vi "IO_Driver18v7.vi"(10 "Inputs":T3, 11 "Reply In":string) -> (0 "Tx Buf Out":string, 2 "Outputs":T2)   [LabVIEW 2024]
uses:
  Control Definitions/Def_Status18v7.ctl
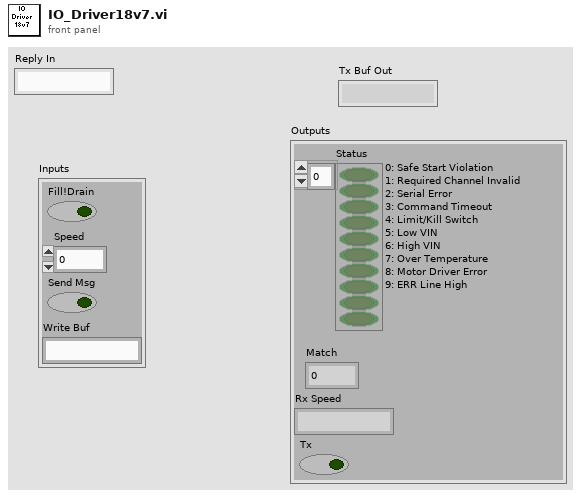
[diagram p1: front panel]
types:
  T1 = typedef "Def_Status18v7.ctl" = bool[]
  T2 = cluster{"Status":T1, "Match":i32, "Rx Speed":string, "Tx":bool}
  T3 = cluster{"Fill!Drain":bool, "Speed":i16, "Send Msg":bool, "Write Buf":string}
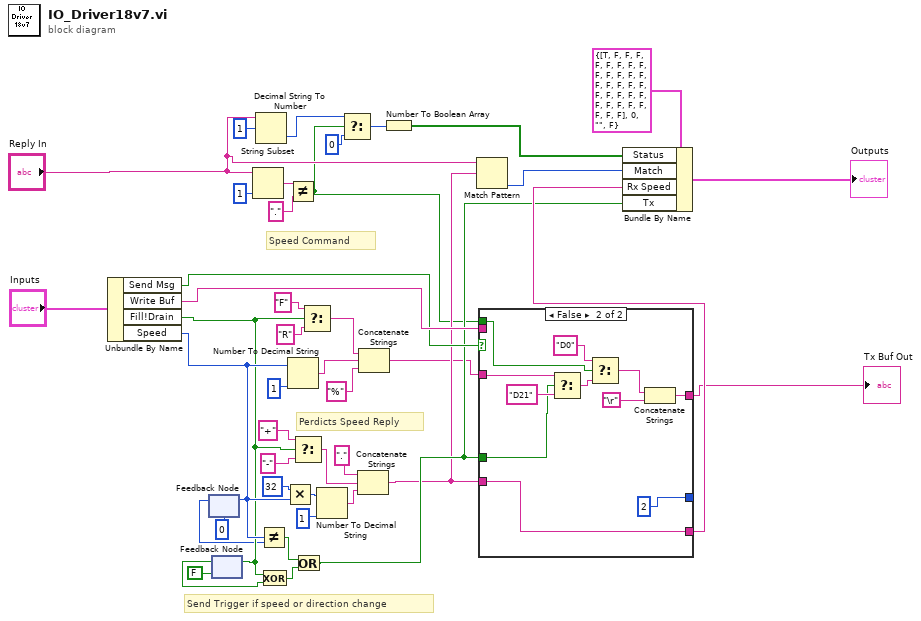
[diagram p0: block diagram]
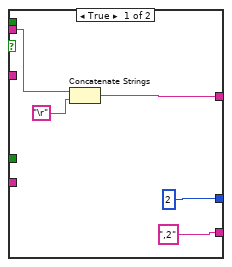
[diagram p2: hidden frame]
diagram:
  # "Send Trigger if speed or direction change"
  # "Speed Command"
  # "Perdicts Speed Reply"
  n1 = Unbundle By Name("Inputs") -> ("Send Msg"=w39:bool, "Write Buf"=w40:string, "Fill!Drain"=w41:bool, "Speed"=w42:i16)
  n2 = feedback #1(i16 0 ("Speed")) -> (w12:i16)
  n3 = feedback-in #1(w42) -> ()
  n4 = feedback #2(FALSE ("Fill!Drain")) -> (w20:bool)
  n5 = feedback-in #2(w41) -> ()
  n6 = String Subset(string="Reply In", length (rest)=1 ("length (rest)")) -> (substring=w25:string)  [unwired: 1 in]
  n7 = Decimal String To Number(string="Reply In", offset=1) -> (number=w28:i32)  [unwired: 1 in, 1 out]
  n8 = Not Equal?(x=w42, y=w12) -> (x != y?=w21:bool)
  n9 = Exclusive Or(1:w20, 2:w41) -> (0:w22:bool)
  n10 = Multiply(x=32, y=w42) -> (x*y=w7:i32)
  n11 = Not Equal?(x=w25, y=".") -> (x != y?=w30:bool)
  n12 = Number To Decimal String(number=w42, width (-)=i16 1) -> (decimal integer string=w17:string)
  n13 = Select(t="+", s=w41, f="-") -> (s? t:f=w9:string)
  n14 = Or(x=w21, y=w22) -> (x .or. y?=w36:bool)
  n15 = Select(t="F", s=w41, f="R") -> (s? t:f=w16:string)
  n16 = Number To Decimal String(number=w7, width (-)=i16 1) -> (decimal integer string=w8:string)
  n17 = Select(t=w28, s=w30, f=0) -> (s? t:f=w27:i32)
  n18 = Concatenate Strings(".", w9, w8) -> (w31:string)
  n19 = Concatenate Strings(w16, w17, "%" ("string")) -> (w1:string)
  n20 = Number To Boolean Array(number=w27) -> (Boolean array=w33:bool[])
  n21 = Match Pattern(string="Reply In", regular expression=w31) -> (offset past match=w35:i32)  [unwired: 1 in, 3 out]
  n22 = case shown="False" w39 {
    tunnel: w30 -> [_ w49]
    tunnel: w1 -> [_ w54]
    tunnel: [w47 w58] -> w2
    tunnel: [2 2] -> _
    tunnel: w31 -> [_ w56]
    tunnel: [",2" w56] -> w43
    tunnel: w36 -> [_ w52]
    tunnel: w40 -> [w44 _]
    frame True {
      n23 = Concatenate Strings(w44, "\r") -> (w47:string)
    }
    frame False {
      n24 = Select(t=w54, s=w52, f="D21" ("write buffer 2")) -> (s? t:f=w51:string)
      n25 = Select(t="D0" ("write buffer 2"), s=w49, f=w51) -> (s? t:f=w55:string)
      n26 = Concatenate Strings(w55, "\r") -> (w58:string)
    }
  }
  "Tx Buf Out" <- w2
  n27 = Bundle By Name(cluster=T2 {"Status"=[TRUE, FALSE, FALSE, FALSE, FALSE, FALSE, FALSE, FALSE, FALSE, FALSE, FALSE, FALSE, FALSE, FALSE, FALSE, FALSE, FALSE, FALSE, FALSE, FALSE, FALSE, FALSE, FALSE, FALSE, FALSE, FALSE, FALSE, FALSE, FALSE, FALSE, FALSE, FALSE], "Match"=0, "Rx Speed"="", "Tx"=FALSE} ("Cluster"), "Status"=w33, "Match"=w35, "Rx Speed"=w43, "Tx"=w36) -> (→"Outputs":T2)
